vi "char_to_float.vi"(1 "index of float":i32, 2 "data input":string) -> (0 "float output":dbl)   [LabVIEW 2020]
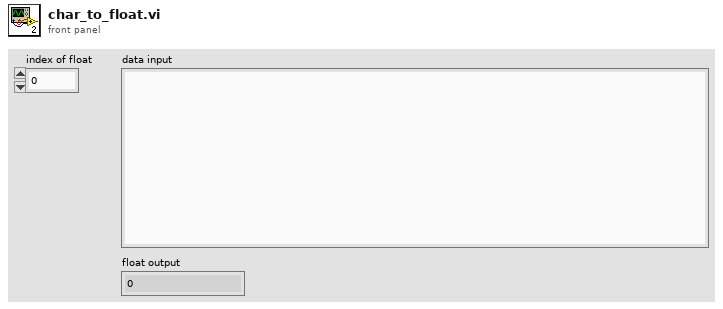
[diagram p1: front panel]
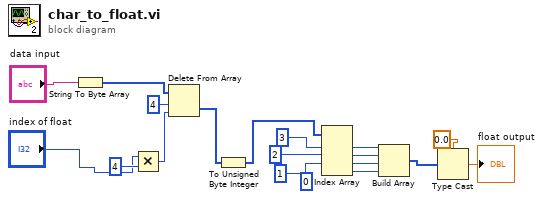
[diagram p0: block diagram]
diagram:
  (unwired) 0 ("index")
  n1 = String To Byte Array(string="data input") -> (unsigned byte array=w15:u8[])
  n2 = Multiply(x="index of float", y=4) -> (x*y=w14:i32)
  n3 = Delete From Array(array=w15, length=4, index=w14) -> (deleted portion=w12:u8[])  [unwired: 1 out]
  n4 = To Unsigned Byte Integer(number=w12) -> (unsigned 8bit integer=w8:u8[])
  n5 = Index Array(array=w8, index #1=3 ("index"), index #2=2 ("index"), index #3=1 ("index")) -> (element #1=w7:u8, element #2=w6:u8, element #3=w5:u8, element #4=w4:u8)  [unwired: 1 in]
  n6 = Build Array(w7, w6, w5, w4) -> (w1:u8[])
  n7 = Type Cast(type=sgl 0.0 ("number"), x=w1) -> (*(type *) &x=→"float output":sgl)
